vi "Get Unitless Values.vi"(8 "error in (no error)":errorcluster, 11 "Analyze Results Energy in":refnum<class "Analyze Results Energy.lvclass">) -> (0 "error out":errorcluster, 2 "UnitLess Values":T1[](array[typedef]), 3 "Analyze Results Energy out":refnum<class "Analyze Results Energy.lvclass">)   [LabVIEW 2020, in "Analyze Results Energy.lvclass"]
uses:
  Analyze Results Energy.lvclass
  Results Base/UnitLessValue.ctl
  Analyze Results Energy.lvclass/Analyze Results Energy.ctl
  Results Base/Analyze Results Base.lvclass
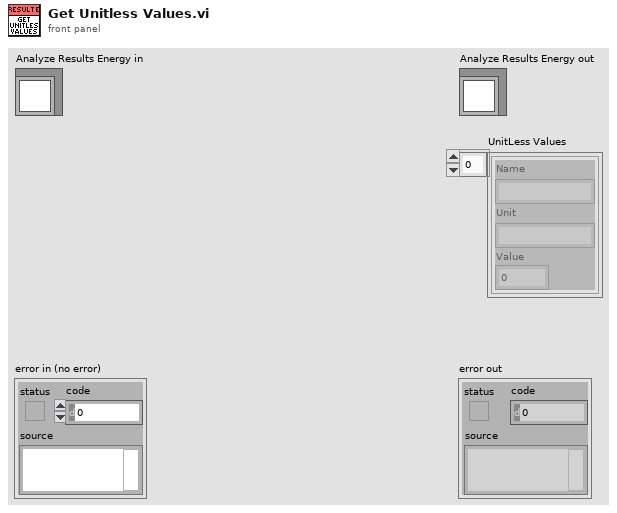
[diagram p1: front panel]
types:
  T1 = typedef "Analyze Results Base.lvclass/UnitLessValue.ctl" = cluster{"Name":string, "Unit":string, "Value":dbl}
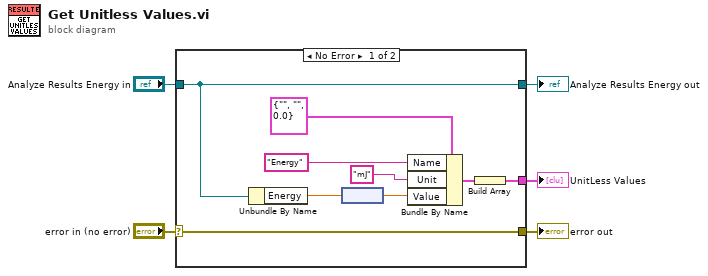
[diagram p0: block diagram]
diagram:
  n1 = case shown="No Error" "error in (no error)" {
    selector: "error in (no error)" -> [w11 w15]
    tunnel: "Analyze Results Energy in" -> [w12 w16]
    tunnel: [w6 _] -> w3
    tunnel: [w12 w16] -> w4
    tunnel: [w11 w15] -> w1
    frame No Error {
      n2 = Unbundle By Name(w12) -> ("Energy"=w10:dbl[unit])
      n3 = node(w10) -> (w8:dbl)
      n4 = Bundle By Name(cluster=T1 {"Name"="", "Unit"="", "Value"=0.0} ("UnitLessValue"), "Name"="Energy", "Unit"="mJ", "Value"=w8) -> (w13:T1)
      n5 = Build Array(w13) -> (w6:T1[])
    }
    frame Error {
    }
  }
  "error out" <- w1
  "Analyze Results Energy out" <- w4
  "UnitLess Values" <- w3
